vi "ComplexExamples.vi"() -> ()   [LabVIEW 2013]
uses:
  TypeDefs/ctl_ExampleComplexCluster.ctl
  TypeDefs/ctl_ElementAndPaddingInfo.ctl
  TypeDefs/ctl_DataElementInfo.ctl
panel:
  out "CalibrationLampInfo.LampType":string
  out "Element and Padding Info (Large Struct2)":T1
  out "Element and Padding Info (Wave Element 2)":T1
  out "Element and Padding Info (Wave Array as Struct1)":T1
  out "Element and Padding Info (Large Struct1)":T1
  out "Array":cluster{"X":i32, "Y":dbl}[](array[cluster])
  in  "#pragma packing directive (0, default) 2":i32=8
  in  "byte order (0:big-endian, network order) 2":T3(ring)=enum."native, host order"
  out "ComplexClusterReturned 2":T4
  out "value":cluster{cluster{"X":i32, "Y":dbl}[]}
  out "ComplexClusterReturned":T4
  in  "byte order (0:big-endian, network order)":T3(ring)=enum."native, host order"
  in  "#pragma packing directive (0, default)":i32=8
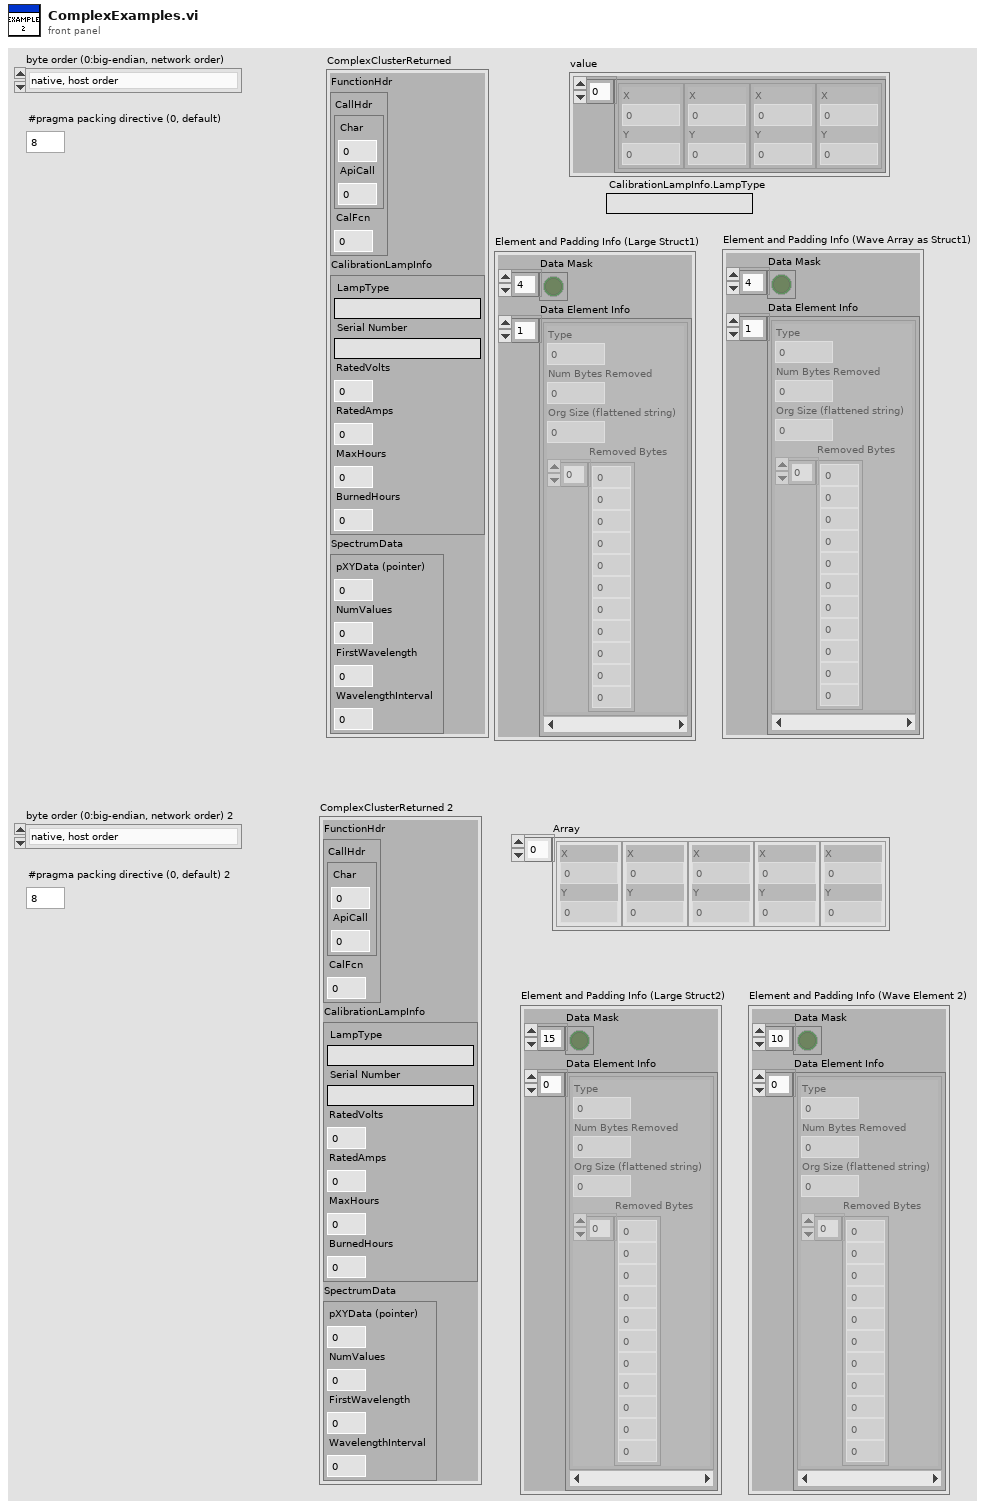
[diagram p1: front panel]
types:
  T1 = typedef "ctl_ElementAndPaddingInfo.ctl" = cluster{"Data Mask":bool[], "Data Element Info":T2[]}
  T2 = typedef "ctl_DataElementInfo.ctl" = cluster{"Type":u16, "Num Bytes Removed":u16, "Org Size (flattened string)":i32, "Removed Bytes":u8[]}
  T3 = enum16{"big-endian, network order", "native, host order", "little-endian"}
  T4 = typedef "ctl_ExampleComplexCluster.ctl" = cluster{"FunctionHdr":cluster{"CallHdr":cluster{"Char":u8, "ApiCall":i32}, "CalFcn":i32}, "CalibrationLampInfo":cluster{"LampType":string, "Serial Number":string, "RatedVolts":dbl, "RatedAmps":dbl, "MaxHours":dbl, "BurnedHours":dbl}, "SpectrumData":cluster{"pXYData (pointer)":i32, "NumValues":i32, "FirstWavelength":u32, "WavelengthInterval":u32}}
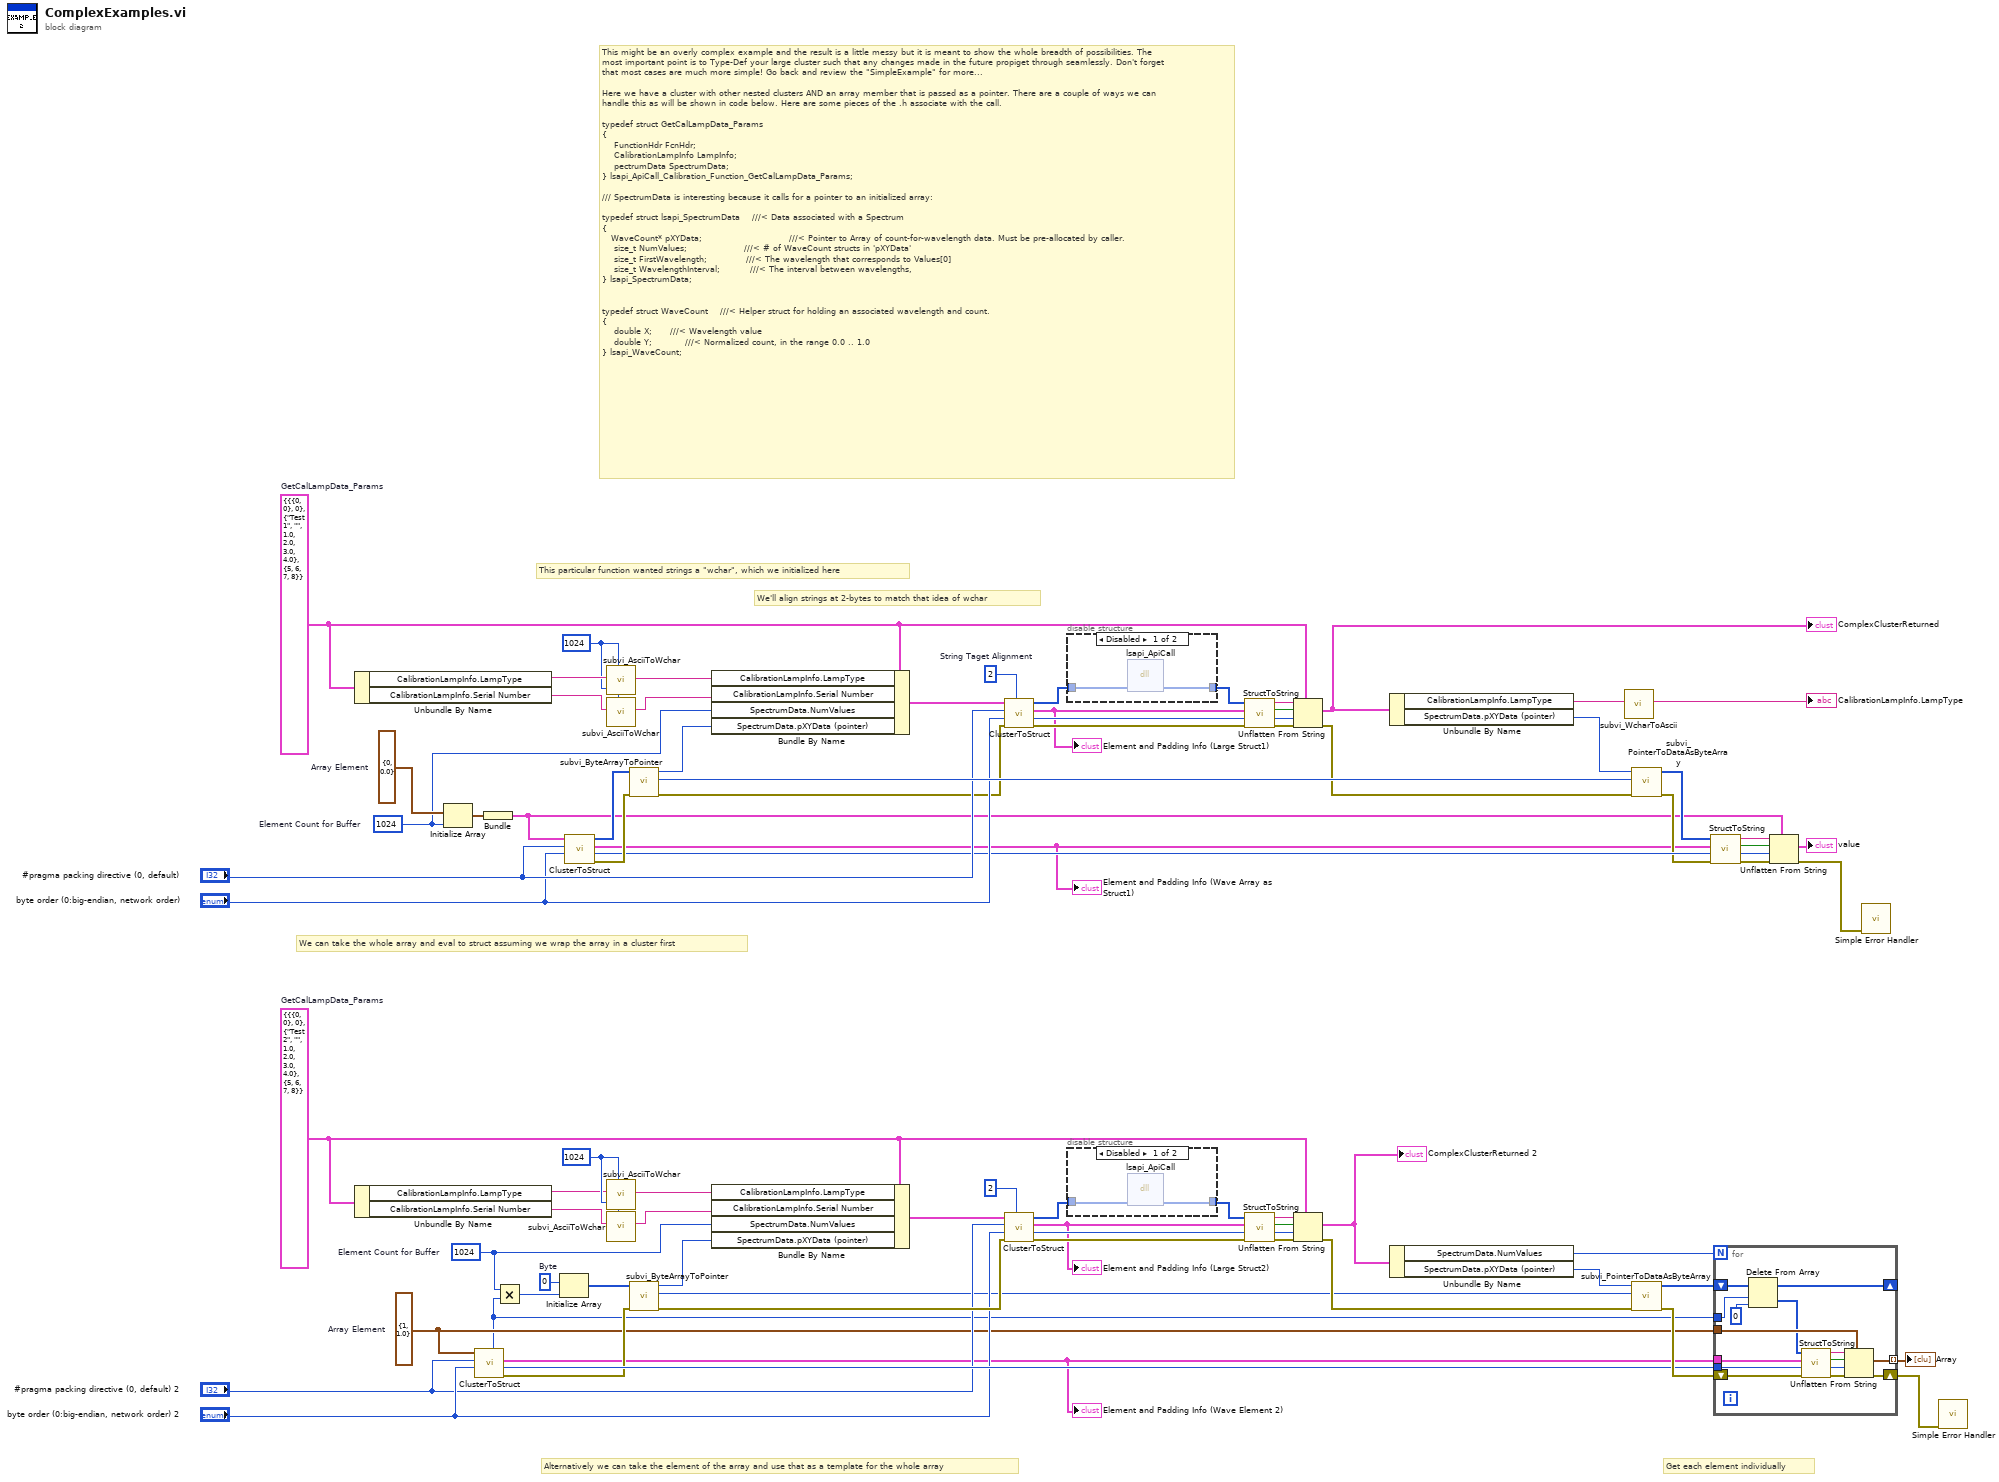
[diagram p0: block diagram]
diagram:
  w12 = u8 0  # Byte
  w15 = cluster{"X":i32, "Y":dbl} {"X"=1, "Y"=1.0}  # Array Element
  w13 = 1024  # Element Count for Buffer
  w19 = 1024 ("Text Buffer Size")
  w37 = T4 {"FunctionHdr"={"CallHdr"={"Char"=0, "ApiCall"=0}, "CalFcn"=0}, "CalibrationLampInfo"={"LampType"="Test2", "Serial Number"="", "RatedVolts"=1.0, "RatedAmps"=2.0, "MaxHours"=3.0, "BurnedHours"=4.0}, "SpectrumData"={"pXYData (pointer)"=5, "NumValues"=6, "FirstWavelength"=7, "WavelengthInterval"=8}}  # GetCalLampData_Params
  w73 = cluster{"X":i32, "Y":dbl} {"X"=0, "Y"=0.0}  # Array Element
  w74 = 2  # String Taget Alignment
  w66 = 1024  # Element Count for Buffer
  w79 = 1024 ("Text Buffer Size")
  w58 = T4 {"FunctionHdr"={"CallHdr"={"Char"=0, "ApiCall"=0}, "CalFcn"=0}, "CalibrationLampInfo"={"LampType"="Test1", "Serial Number"="", "RatedVolts"=1.0, "RatedAmps"=2.0, "MaxHours"=3.0, "BurnedHours"=4.0}, "SpectrumData"={"pXYData (pointer)"=5, "NumValues"=6, "FirstWavelength"=7, "WavelengthInterval"=8}}  # GetCalLampData_Params
  # "This might be an overly complex example and the result is a little messy but it is meant to show the whole breadth of possibilities. The most important point is to Type-Def your large cluster such that any changes made in the future propiget through seamlessly. Don't forget that most cases are much more simple! Go back and review the \"SimpleExample\" for more...\n\nHere we have a cluster with other nested clusters AND an array member that is passed as a pointer. There are a couple of ways we can handle this as will be shown in code below. Here are some pieces of the .h associate with the call.\n\ntypedef struct GetCalLampData_Params \n{\n    FunctionHdr FcnHdr;            \n    CalibrationLampInfo LampInfo;    \n    pectrumData SpectrumData;            \n} lsapi_ApiCall_Calibration_Function_GetCalLampData_Params;\n\n/// SpectrumData is interesting because it calls for a pointer to an initialized array:\n\ntypedef struct lsapi_SpectrumData    ///< Data associated with a Spectrum\n{\n   WaveCount* pXYData;                             ///< Pointer to Array of count-for-wavelength data. Must be pre-allocated by caller.\n    size_t NumValues;                   ///< # of WaveCount structs in 'pXYData'\n    size_t FirstWavelength;             ///< The wavelength that corresponds to Values[0]\n    size_t WavelengthInterval;          ///< The interval between wavelengths,\n} lsapi_SpectrumData;\n\n\ntypedef struct WaveCount    ///< Helper struct for holding an associated wavelength and count.\n{\n    double X;      ///< Wavelength value\n    double Y;           ///< Normalized count, in the range 0.0 .. 1.0\n} lsapi_WaveCount;"
  # "Get each element individually"
  # "Alternatively we can take the element of the array and use that as a template for the whole array"
  # "We can take the whole array and eval to struct assuming we wrap the array in a cluster first"
  # "We'll align strings at 2-bytes to match that idea of wchar"
  # "This particular function wanted strings a \"wchar\", which we initialized here"
  n1 = Unbundle By Name(w58) -> ("CalibrationLampInfo.LampType"=w82:string, "CalibrationLampInfo.Serial Number"=w81:string)
  n2 = Unbundle By Name(w37) -> ("CalibrationLampInfo.LampType"=w16:string, "CalibrationLampInfo.Serial Number"=w17:string)
  n3 = Initialize Array(w73, w66) -> (w46:cluster{"X":i32, "Y":dbl}[])
  n4 = call "ClusterToStruct.vi"("byte order (1, host order checking)"="byte order (0:big-endian, network order) 2", "#pragma packing directive (0, default)"="#pragma packing directive (0, default) 2", "LV Cluster"=w15) -> ("error out"=w32:errorcluster, "byte order Used"=w41:T3, "Element and Padding Info"=w3:T1, "Struct Size"=w9:i32)  [unwired: 4 in, 1 out]
  "Element and Padding Info (Wave Element 2)" <- w3
  n5 = Bundle(w46) -> (w47:cluster{cluster{"X":i32, "Y":dbl}[]})  [unwired: 1 in]
  n6 = Multiply(x=w13, y=w9) -> (x*y=w14:i32)
  n7 = Initialize Array(w12, w14) -> (w11:u8[])
  n8 = call "ClusterToStruct.vi"("byte order (1, host order checking)"="byte order (0:big-endian, network order)", "#pragma packing directive (0, default)"="#pragma packing directive (0, default)", "LV Cluster"=w47) -> ("error out"=w63:errorcluster, "byte order Used"=w54:T3, "Element and Padding Info"=w5:T1, "Cluster Data as Byte Array Out"=w69:u8[])  [unwired: 4 in, 1 out]
  "Element and Padding Info (Wave Array as Struct1)" <- w5
  n9 = call "subvi_AsciiToWchar.vi"("Text Buffer Size"=w79, "ASCII string IN"=w82) -> ("Flattened wchar"=w78:string)  [unwired: 8 in, 1 out]
  n10 = call "subvi_AsciiToWchar.vi"("Text Buffer Size"=w79, "ASCII string IN"=w81) -> ("Flattened wchar"=w80:string)  [unwired: 8 in, 1 out]
  n11 = call "subvi_AsciiToWchar.vi"("Text Buffer Size"=w19, "ASCII string IN"=w16) -> ("Flattened wchar"=w20:string)  [unwired: 8 in, 1 out]
  n12 = call "subvi_AsciiToWchar.vi"("Text Buffer Size"=w19, "ASCII string IN"=w17) -> ("Flattened wchar"=w18:string)  [unwired: 8 in, 1 out]
  n13 = call "subvi_ByteArrayToPointer.vi"("error in (no error)"=w63, "Byte Array In"=w69) -> ("error out"=w62:errorcluster, "Size"=w77:i32, "Pointer"=w76:i32)  [unwired: 7 in]
  n14 = call "subvi_ByteArrayToPointer.vi"("error in (no error)"=w32, "Byte Array In"=w11) -> ("error out"=w33:errorcluster, "Size"=w21:i32, "Pointer"=w22:i32)  [unwired: 7 in]
  n15 = Bundle By Name(cluster=w58, "CalibrationLampInfo.LampType"=w78, "CalibrationLampInfo.Serial Number"=w80, "SpectrumData.NumValues"=w66, "SpectrumData.pXYData (pointer)"=w76) -> (w75:T4)
  n16 = Bundle By Name(cluster=w37, "CalibrationLampInfo.LampType"=w20, "CalibrationLampInfo.Serial Number"=w18, "SpectrumData.NumValues"=w13, "SpectrumData.pXYData (pointer)"=w22) -> (w23:T4)
  n17 = call "ClusterToStruct.vi"("String Taget Alignment (1)"=w74, "error in (no error)"=w62, "byte order (1, host order checking)"="byte order (0:big-endian, network order)", "#pragma packing directive (0, default)"="#pragma packing directive (0, default)", "LV Cluster"=w75) -> ("error out"=w65:errorcluster, "byte order Used"=w70:T3, "Element and Padding Info"=w6:T1, "Cluster Data as Byte Array Out"=w72:u8[])  [unwired: 2 in, 1 out]
  "Element and Padding Info (Large Struct1)" <- w6
  n18 = call "ClusterToStruct.vi"("String Taget Alignment (1)"=2, "error in (no error)"=w33, "byte order (1, host order checking)"="byte order (0:big-endian, network order) 2", "#pragma packing directive (0, default)"="#pragma packing directive (0, default) 2", "LV Cluster"=w23) -> ("error out"=w30:errorcluster, "byte order Used"=w27:T3, "Element and Padding Info"=w4:T1, "Cluster Data as Byte Array Out"=w25:u8[])  [unwired: 2 in, 1 out]
  "Element and Padding Info (Large Struct2)" <- w4
  n19 = disable-structure shown="Disabled" {
    disable-tunnel: w72 -> [w84 w85]
    disable-tunnel: [w83 w85] -> w71
    frame Disabled {
      n20 = dll-call lib="?" fn="lsapi_ApiCall" label="Call Library Function Node"("ApiCallHdr"=w84) -> ("ApiCallHdr"=w83:u8[])  [unwired: 4 in, 2 out]
    }
    frame Enabled {
    }
  }
  n21 = disable-structure shown="Disabled" {
    disable-tunnel: w25 -> [w87 w88]
    disable-tunnel: [w86 w88] -> w26
    frame Disabled {
      n22 = dll-call lib="?" fn="lsapi_ApiCall" label="Call Library Function Node"("ApiCallHdr"=w87) -> ("ApiCallHdr"=w86:u8[])  [unwired: 4 in, 2 out]
    }
    frame Enabled {
    }
  }
  n23 = call "StructToString.vi"("error in (no error)"=w65, "byte order"=w70, "Element and Padding Info"=w6, "Data as Unsigned Byte Array (with padding)"=w71) -> ("error out"=w64:errorcluster, "byte order (0:big-endian, network order) 2"=w59:T3, "Size Included (Always F)"=w60:bool, "Data As String for Unflatten Function"=w61:string)  [unwired: 4 in]
  n24 = call "StructToString.vi"("error in (no error)"=w30, "byte order"=w27, "Element and Padding Info"=w4, "Data as Unsigned Byte Array (with padding)"=w26) -> ("error out"=w31:errorcluster, "byte order (0:big-endian, network order) 2"=w36:T3, "Size Included (Always F)"=w35:bool, "Data As String for Unflatten Function"=w34:string)  [unwired: 4 in]
  n25 = Unflatten From String(type=w58, binary string=w61, data includes array or string size? (T)=w60, byte order (0:big-endian, network order)=w59, error in (no error)=w64) -> (value=w57:T4, error out=w53:errorcluster)  [unwired: 1 out]
  "ComplexClusterReturned" <- w57
  n26 = Unflatten From String(type=w37, binary string=w34, data includes array or string size? (T)=w35, byte order (0:big-endian, network order)=w36, error in (no error)=w31) -> (value=w38:T4, error out=w42:errorcluster)  [unwired: 1 out]
  "ComplexClusterReturned 2" <- w38
  n27 = Unbundle By Name(w57) -> ("CalibrationLampInfo.LampType"=w2:string, "SpectrumData.pXYData (pointer)"=w56:i32)
  n28 = Unbundle By Name(w38) -> ("SpectrumData.NumValues"=w10:i32, "SpectrumData.pXYData (pointer)"=w39:i32)
  n29 = call "subvi_WcharToAscii.vi"("Flattened whar IN"=w2) -> ("ASCII"=→"CalibrationLampInfo.LampType":string)  [unwired: 10 in]
  n30 = call "subvi_PointerToDataAsByteArray.vi"("error in (no error)"=w53, "Size"=w77, "Pointer"=w56) -> ("error out"=w52:errorcluster, "Byte Array Out"=w55:u8[])  [unwired: 7 in]
  n31 = call "subvi_PointerToDataAsByteArray.vi"("error in (no error)"=w42, "Size"=w21, "Pointer"=w39) -> ("error out"=w43:errorcluster, "Byte Array Out"=w40:u8[])  [unwired: 7 in]
  n32 = call "StructToString.vi"("error in (no error)"=w52, "byte order"=w54, "Element and Padding Info"=w5, "Data as Unsigned Byte Array (with padding)"=w55) -> ("error out"=w49:errorcluster, "byte order (0:big-endian, network order) 2"=w50:T3, "Size Included (Always F)"=w48:bool, "Data As String for Unflatten Function"=w51:string)  [unwired: 4 in]
  n33 = for {
    N: w10 -> [_]
    tunnel: [w103] -> w8 mode=indexing
    tunnel: w41 -> [w97]
    tunnel: w3 -> [w96]
    tunnel: w15 -> [w95]
    shift-right: [w94] -> w7
    shift-left: w43 -> [w98]
    shift-right: [w89] -> _
    shift-left: w40 -> [w93]
    tunnel: w9 -> [w91]
    n34 = Delete From Array(array=w93, length=w91, index=0) -> (deleted portion=w90:u8[], array with subset deleted=w89:u8[])
    n35 = call "StructToString.vi"("error in (no error)"=w98, "byte order"=w97, "Element and Padding Info"=w96, "Data as Unsigned Byte Array (with padding)"=w90) -> ("error out"=w101:errorcluster, "byte order (0:big-endian, network order) 2"=w100:T3, "Size Included (Always F)"=w102:bool, "Data As String for Unflatten Function"=w99:string)  [unwired: 4 in]
    n36 = Unflatten From String(type=w95, binary string=w99, data includes array or string size? (T)=w102, byte order (0:big-endian, network order)=w100, error in (no error)=w101) -> (value=w103:cluster{"X":i32, "Y":dbl}, error out=w94:errorcluster)  [unwired: 1 out]
  }
  "Array" <- w8
  n37 = Unflatten From String(type=w47, binary string=w51, data includes array or string size? (T)=w48, byte order (0:big-endian, network order)=w50, error in (no error)=w49) -> (value=→"value":cluster{cluster{"X":i32, "Y":dbl}[]}, error out=w44:errorcluster)  [unwired: 1 out]
  n38 = call <vilib>:"Simple Error Handler.vi"("error in (no error)"=w44) -> ()  [unwired: 4 in, 5 out]
  n39 = call <vilib>:"Simple Error Handler.vi"("error in (no error)"=w7) -> ()  [unwired: 4 in, 5 out]
